vi "FormatDefor.vi"(6 "UnidadesD":u16(ring) caption="Unidades" items=["mm", "inch"], 8 "ValorIn":dbl, 9 "CaptadorD":u16(ring) caption="Captador" items=["Deformación"], 11 "ResoExten":i8(ring) caption="Resolució" items=["0.1", "0.2", "0.5", "0.01", "0.02", "0.05", "0.001", "0.002", "0.005"]) -> (0 "ValorOut":dbl, 3 "NDecimals":u8)   [LabVIEW 2017]
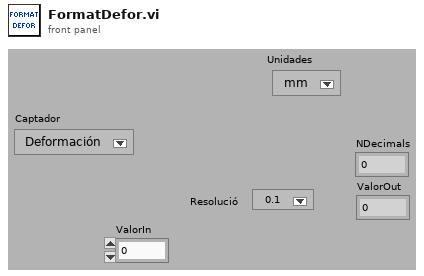
[diagram p1: front panel]
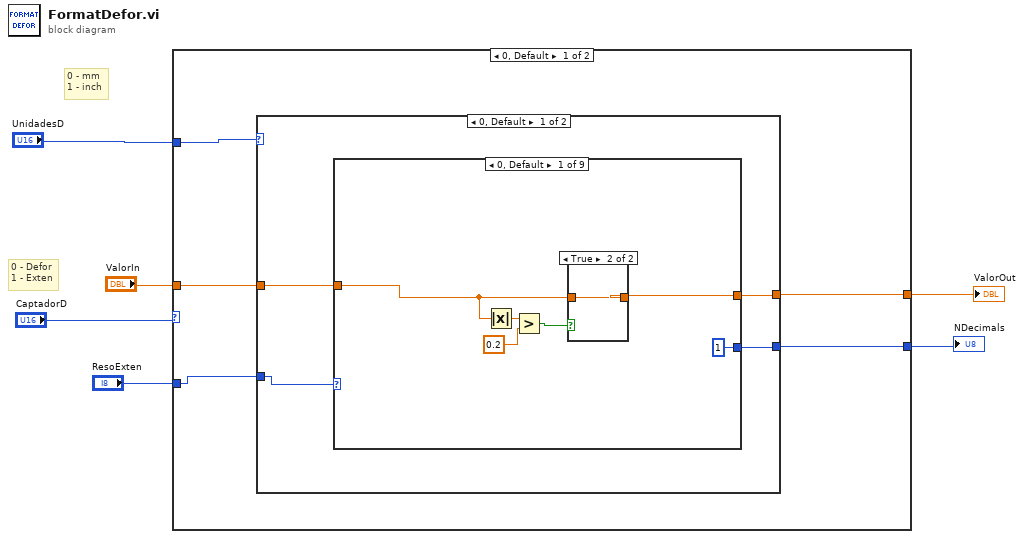
[diagram p0: block diagram]
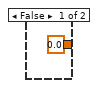
[diagram p2: hidden frame]
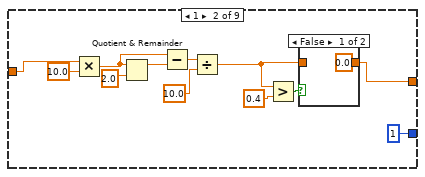
[diagram p3: hidden frame]
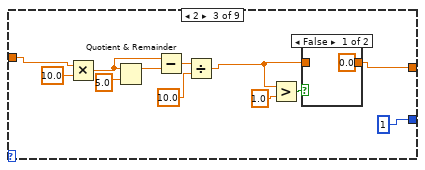
[diagram p5: hidden frame]
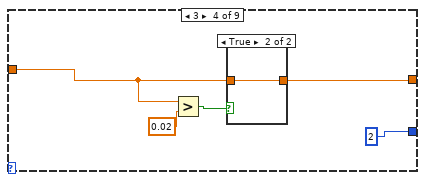
[diagram p7: hidden frame]
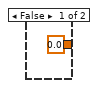
[diagram p8: hidden frame]
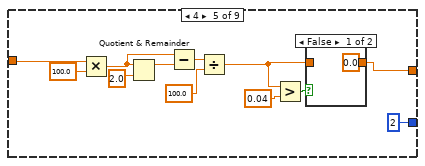
[diagram p9: hidden frame]
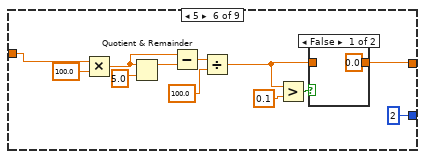
[diagram p11: hidden frame]
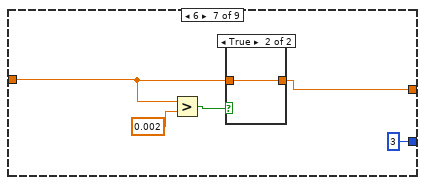
[diagram p13: hidden frame]
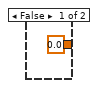
[diagram p14: hidden frame]
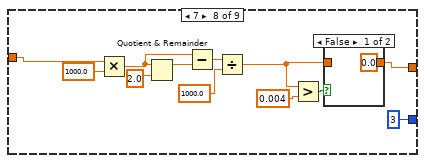
[diagram p15: hidden frame]
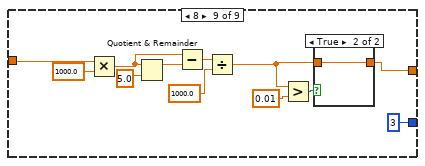
[diagram p17: hidden frame]
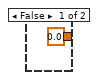
[diagram p18: hidden frame]
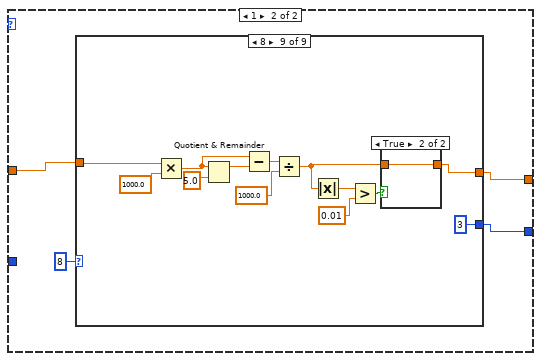
[diagram p19: hidden frame]
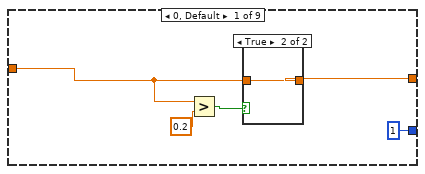
[diagram p20: hidden frame]
diagram:
  # "0 - Defor\n1 - Exten"
  # "0 - mm\n1 - inch"
  n1 = case shown="0, Default" "CaptadorD" {
    tunnel: "ResoExten" -> [w9 w236]
    tunnel: "ValorIn" -> [w10 w235]
    tunnel: [w8 w234] -> w4
    tunnel: [w7 w233] -> w3
    tunnel: "UnidadesD" -> [w11 w232]
    frame 0, Default {
      n2 = case shown="0, Default" w11 {
        tunnel: w10 -> [w13 w125]
        tunnel: w9 -> [w12 _]
        tunnel: [w14 w124] -> w8
        tunnel: [w15 w123] -> w7
        frame 0, Default {
          n3 = case shown="0, Default" w12 {
            tunnel: w13 -> [w18 w25 w40 w54 w61 w74 w89 w95 w110]
            tunnel: [w19 w26 w39 w53 w60 w75 w88 w96 w109] -> w15
            tunnel: [1 ("NDecimals") 1 ("NDecimals") 1 2 ("NDecimals") 2 ("NDecimals") 2 ("NDecimals") 3 ("NDecimals") 3 ("NDecimals") 3 ("NDecimals")] -> w14
            frame 0, Default {
              n4 = Absolute Value(x=w18) -> (abs(x)=w16:dbl)
              n5 = Greater?(x=w16, y=0.2) -> (0:w20:bool)
              n6 = case shown="True" w20 {
                tunnel: w18 -> [_ w23]
                tunnel: [0.0 w23] -> w19
                frame False {
                }
                frame True {
                }
              }
            }
            frame 1 {
              n7 = Multiply(x=w25, y=10.0) -> (x*y=w32:dbl)
              n8 = Quotient & Remainder(x=w32, y=2.0) -> (x-y*floor(x/y)=w33:dbl)  [unwired: 1 out]
              n9 = Subtract(x=w32, y=w33) -> (x-y=w31:dbl)
              n10 = Divide(x=w31, y=10.0) -> (x/y=w27:dbl)
              n11 = Greater?(x=w27, y=0.4) -> (0:w29:bool)
              n12 = case shown="False" w29 {
                tunnel: w27 -> [_ w37]
                tunnel: [0.0 w37] -> w26
                frame False {
                }
                frame True {
                }
              }
            }
            frame 2 {
              n13 = Multiply(x=w40, y=10.0) -> (x*y=w46:dbl)
              n14 = Quotient & Remainder(x=w46, y=5.0) -> (x-y*floor(x/y)=w47:dbl)  [unwired: 1 out]
              n15 = Subtract(x=w46, y=w47) -> (x-y=w45:dbl)
              n16 = Divide(x=w45, y=10.0) -> (x/y=w41:dbl)
              n17 = Greater?(x=w41, y=1.0) -> (0:w43:bool)
              n18 = case shown="False" w43 {
                tunnel: w41 -> [_ w51]
                tunnel: [0.0 w51] -> w39
                frame False {
                }
                frame True {
                }
              }
            }
            frame 3 {
              n19 = Greater?(x=w54, y=0.02) -> (0:w55:bool)
              n20 = case shown="True" w55 {
                tunnel: w54 -> [_ w58]
                tunnel: [0.0 w58] -> w53
                frame False {
                }
                frame True {
                }
              }
            }
            frame 4 {
              n21 = Multiply(x=w61, y=100.0) -> (x*y=w67:dbl)
              n22 = Quotient & Remainder(x=w67, y=2.0) -> (x-y*floor(x/y)=w68:dbl)  [unwired: 1 out]
              n23 = Subtract(x=w67, y=w68) -> (x-y=w66:dbl)
              n24 = Divide(x=w66, y=100.0) -> (x/y=w62:dbl)
              n25 = Greater?(x=w62, y=0.04) -> (0:w64:bool)
              n26 = case shown="False" w64 {
                tunnel: w62 -> [_ w72]
                tunnel: [0.0 w72] -> w60
                frame False {
                }
                frame True {
                }
              }
            }
            frame 5 {
              n27 = Multiply(x=w74, y=100.0) -> (x*y=w81:dbl)
              n28 = Quotient & Remainder(x=w81, y=5.0) -> (x-y*floor(x/y)=w82:dbl)  [unwired: 1 out]
              n29 = Subtract(x=w81, y=w82) -> (x-y=w80:dbl)
              n30 = Divide(x=w80, y=100.0) -> (x/y=w76:dbl)
              n31 = Greater?(x=w76, y=0.1) -> (0:w78:bool)
              n32 = case shown="False" w78 {
                tunnel: w76 -> [_ w86]
                tunnel: [0.0 w86] -> w75
                frame False {
                }
                frame True {
                }
              }
            }
            frame 6 {
              n33 = Greater?(x=w89, y=0.002) -> (0:w90:bool)
              n34 = case shown="True" w90 {
                tunnel: w89 -> [_ w93]
                tunnel: [0.0 w93] -> w88
                frame False {
                }
                frame True {
                }
              }
            }
            frame 7 {
              n35 = Multiply(x=w95, y=1000.0) -> (x*y=w102:dbl)
              n36 = Quotient & Remainder(x=w102, y=2.0) -> (x-y*floor(x/y)=w103:dbl)  [unwired: 1 out]
              n37 = Subtract(x=w102, y=w103) -> (x-y=w101:dbl)
              n38 = Divide(x=w101, y=1000.0) -> (x/y=w97:dbl)
              n39 = Greater?(x=w97, y=0.004) -> (0:w99:bool)
              n40 = case shown="False" w99 {
                tunnel: w97 -> [_ w107]
                tunnel: [0.0 w107] -> w96
                frame False {
                }
                frame True {
                }
              }
            }
            frame 8 {
              n41 = Multiply(x=w110, y=1000.0) -> (x*y=w116:dbl)
              n42 = Quotient & Remainder(x=w116, y=5.0) -> (x-y*floor(x/y)=w117:dbl)  [unwired: 1 out]
              n43 = Subtract(x=w116, y=w117) -> (x-y=w115:dbl)
              n44 = Divide(x=w115, y=1000.0) -> (x/y=w111:dbl)
              n45 = Greater?(x=w111, y=0.01) -> (0:w113:bool)
              n46 = case shown="True" w113 {
                tunnel: w111 -> [_ w121]
                tunnel: [0.0 w121] -> w109
                frame False {
                }
                frame True {
                }
              }
            }
          }
        }
        frame 1 {
          n47 = case shown="8" i8 8 ("ResoExten") {
            tunnel: w125 -> [w127 w134 w149 w163 w170 w183 w198 w204 w220]
            tunnel: [w128 w135 w148 w162 w169 w184 w197 w205 w219] -> w123
            tunnel: [1 ("NDecimals") 1 ("NDecimals") 1 2 ("NDecimals") 2 ("NDecimals") 2 ("NDecimals") 3 ("NDecimals") 3 ("NDecimals") 3 ("NDecimals")] -> w124
            frame 0, Default {
              n48 = Greater?(x=w127, y=0.2) -> (0:w129:bool)
              n49 = case shown="True" w129 {
                tunnel: w127 -> [_ w132]
                tunnel: [0.0 w132] -> w128
                frame False {
                }
                frame True {
                }
              }
            }
            frame 1 {
              n50 = Multiply(x=w134, y=10.0) -> (x*y=w141:dbl)
              n51 = Quotient & Remainder(x=w141, y=2.0) -> (x-y*floor(x/y)=w142:dbl)  [unwired: 1 out]
              n52 = Subtract(x=w141, y=w142) -> (x-y=w140:dbl)
              n53 = Divide(x=w140, y=10.0) -> (x/y=w136:dbl)
              n54 = Greater?(x=w136, y=0.4) -> (0:w138:bool)
              n55 = case shown="False" w138 {
                tunnel: w136 -> [_ w146]
                tunnel: [0.0 w146] -> w135
                frame False {
                }
                frame True {
                }
              }
            }
            frame 2 {
              n56 = Multiply(x=w149, y=10.0) -> (x*y=w155:dbl)
              n57 = Quotient & Remainder(x=w155, y=5.0) -> (x-y*floor(x/y)=w156:dbl)  [unwired: 1 out]
              n58 = Subtract(x=w155, y=w156) -> (x-y=w154:dbl)
              n59 = Divide(x=w154, y=10.0) -> (x/y=w150:dbl)
              n60 = Greater?(x=w150, y=1.0) -> (0:w152:bool)
              n61 = case shown="False" w152 {
                tunnel: w150 -> [_ w160]
                tunnel: [0.0 w160] -> w148
                frame False {
                }
                frame True {
                }
              }
            }
            frame 3 {
              n62 = Greater?(x=w163, y=0.02) -> (0:w164:bool)
              n63 = case shown="True" w164 {
                tunnel: w163 -> [_ w167]
                tunnel: [0.0 w167] -> w162
                frame False {
                }
                frame True {
                }
              }
            }
            frame 4 {
              n64 = Multiply(x=w170, y=100.0) -> (x*y=w176:dbl)
              n65 = Quotient & Remainder(x=w176, y=2.0) -> (x-y*floor(x/y)=w177:dbl)  [unwired: 1 out]
              n66 = Subtract(x=w176, y=w177) -> (x-y=w175:dbl)
              n67 = Divide(x=w175, y=100.0) -> (x/y=w171:dbl)
              n68 = Greater?(x=w171, y=0.04) -> (0:w173:bool)
              n69 = case shown="False" w173 {
                tunnel: w171 -> [_ w181]
                tunnel: [0.0 w181] -> w169
                frame False {
                }
                frame True {
                }
              }
            }
            frame 5 {
              n70 = Multiply(x=w183, y=100.0) -> (x*y=w190:dbl)
              n71 = Quotient & Remainder(x=w190, y=5.0) -> (x-y*floor(x/y)=w191:dbl)  [unwired: 1 out]
              n72 = Subtract(x=w190, y=w191) -> (x-y=w189:dbl)
              n73 = Divide(x=w189, y=100.0) -> (x/y=w185:dbl)
              n74 = Greater?(x=w185, y=0.1) -> (0:w187:bool)
              n75 = case shown="False" w187 {
                tunnel: w185 -> [_ w195]
                tunnel: [0.0 w195] -> w184
                frame False {
                }
                frame True {
                }
              }
            }
            frame 6 {
              n76 = Greater?(x=w198, y=0.002) -> (0:w199:bool)
              n77 = case shown="True" w199 {
                tunnel: w198 -> [_ w202]
                tunnel: [0.0 w202] -> w197
                frame False {
                }
                frame True {
                }
              }
            }
            frame 7 {
              n78 = Multiply(x=w204, y=1000.0) -> (x*y=w211:dbl)
              n79 = Quotient & Remainder(x=w211, y=2.0) -> (x-y*floor(x/y)=w212:dbl)  [unwired: 1 out]
              n80 = Subtract(x=w211, y=w212) -> (x-y=w210:dbl)
              n81 = Divide(x=w210, y=1000.0) -> (x/y=w206:dbl)
              n82 = Greater?(x=w206, y=0.004) -> (0:w208:bool)
              n83 = case shown="False" w208 {
                tunnel: w206 -> [_ w216]
                tunnel: [0.0 w216] -> w205
                frame False {
                }
                frame True {
                }
              }
            }
            frame 8 {
              n84 = Multiply(x=w220, y=1000.0) -> (x*y=w226:dbl)
              n85 = Quotient & Remainder(x=w226, y=5.0) -> (x-y*floor(x/y)=w227:dbl)  [unwired: 1 out]
              n86 = Subtract(x=w226, y=w227) -> (x-y=w225:dbl)
              n87 = Divide(x=w225, y=1000.0) -> (x/y=w221:dbl)
              n88 = Absolute Value(x=w221) -> (abs(x)=w217:dbl)
              n89 = Greater?(x=w217, y=0.01) -> (0:w223:bool)
              n90 = case shown="True" w223 {
                tunnel: w221 -> [_ w231]
                tunnel: [0.0 w231] -> w219
                frame False {
                }
                frame True {
                }
              }
            }
          }
        }
      }
    }
    frame 1 {
      n91 = case shown="1" w232 {
        tunnel: w236 -> [w238 _]
        tunnel: w235 -> [w237 w358]
        tunnel: [w239 w357] -> w234
        tunnel: [w240 w356] -> w233
        frame 0, Default {
          n92 = case shown="8" w238 {
            tunnel: [w244 w252 w267 w282 w290 w305 w320 w328 w343] -> w240
            tunnel: [1 ("NDecimals") 1 ("NDecimals") 1 2 ("NDecimals") 2 ("NDecimals") 2 ("NDecimals") 3 ("NDecimals") 3 ("NDecimals") 3 ("NDecimals")] -> w239
            tunnel: w237 -> [w242 w250 w265 w280 w288 w303 w318 w326 w341]
            frame 0, Default {
              n93 = Absolute Value(x=w242) -> (abs(x)=w241:dbl)
              n94 = Greater?(x=w241, y=0.2) -> (0:w245:bool)
              n95 = case shown="True" w245 {
                tunnel: w242 -> [_ w248]
                tunnel: [0.0 w248] -> w244
                frame False {
                }
                frame True {
                }
              }
            }
            frame 1 {
              n96 = Multiply(x=w250, y=10.0) -> (x*y=w258:dbl)
              n97 = Quotient & Remainder(x=w258, y=2.0) -> (x-y*floor(x/y)=w259:dbl)  [unwired: 1 out]
              n98 = Subtract(x=w258, y=w259) -> (x-y=w257:dbl)
              n99 = Divide(x=w257, y=10.0) -> (x/y=w253:dbl)
              n100 = Absolute Value(x=w253) -> (abs(x)=w249:dbl)
              n101 = Greater?(x=w249, y=0.4) -> (0:w255:bool)
              n102 = case shown="False" w255 {
                tunnel: w253 -> [_ w263]
                tunnel: [0.0 w263] -> w252
                frame False {
                }
                frame True {
                }
              }
            }
            frame 2 {
              n103 = Multiply(x=w265, y=10.0) -> (x*y=w273:dbl)
              n104 = Quotient & Remainder(x=w273, y=5.0) -> (x-y*floor(x/y)=w274:dbl)  [unwired: 1 out]
              n105 = Subtract(x=w273, y=w274) -> (x-y=w272:dbl)
              n106 = Divide(x=w272, y=10.0) -> (x/y=w268:dbl)
              n107 = Absolute Value(x=w268) -> (abs(x)=w264:dbl)
              n108 = Greater?(x=w264, y=1.0) -> (0:w270:bool)
              n109 = case shown="False" w270 {
                tunnel: w268 -> [_ w278]
                tunnel: [0.0 w278] -> w267
                frame False {
                }
                frame True {
                }
              }
            }
            frame 3 {
              n110 = Absolute Value(x=w280) -> (abs(x)=w279:dbl)
              n111 = Greater?(x=w279, y=0.02) -> (0:w283:bool)
              n112 = case shown="True" w283 {
                tunnel: w280 -> [_ w286]
                tunnel: [0.0 w286] -> w282
                frame False {
                }
                frame True {
                }
              }
            }
            frame 4 {
              n113 = Multiply(x=w288, y=100.0) -> (x*y=w296:dbl)
              n114 = Quotient & Remainder(x=w296, y=2.0) -> (x-y*floor(x/y)=w297:dbl)  [unwired: 1 out]
              n115 = Subtract(x=w296, y=w297) -> (x-y=w295:dbl)
              n116 = Divide(x=w295, y=100.0) -> (x/y=w291:dbl)
              n117 = Absolute Value(x=w291) -> (abs(x)=w287:dbl)
              n118 = Greater?(x=w287, y=0.04) -> (0:w293:bool)
              n119 = case shown="False" w293 {
                tunnel: w291 -> [_ w301]
                tunnel: [0.0 w301] -> w290
                frame False {
                }
                frame True {
                }
              }
            }
            frame 5 {
              n120 = Multiply(x=w303, y=100.0) -> (x*y=w311:dbl)
              n121 = Quotient & Remainder(x=w311, y=5.0) -> (x-y*floor(x/y)=w312:dbl)  [unwired: 1 out]
              n122 = Subtract(x=w311, y=w312) -> (x-y=w310:dbl)
              n123 = Divide(x=w310, y=100.0) -> (x/y=w306:dbl)
              n124 = Absolute Value(x=w306) -> (abs(x)=w302:dbl)
              n125 = Greater?(x=w302, y=0.1) -> (0:w308:bool)
              n126 = case shown="False" w308 {
                tunnel: w306 -> [_ w316]
                tunnel: [0.0 w316] -> w305
                frame False {
                }
                frame True {
                }
              }
            }
            frame 6 {
              n127 = Absolute Value(x=w318) -> (abs(x)=w317:dbl)
              n128 = Greater?(x=w317, y=0.002) -> (0:w321:bool)
              n129 = case shown="True" w321 {
                tunnel: w318 -> [_ w324]
                tunnel: [0.0 w324] -> w320
                frame False {
                }
                frame True {
                }
              }
            }
            frame 7 {
              n130 = Multiply(x=w326, y=1000.0) -> (x*y=w334:dbl)
              n131 = Quotient & Remainder(x=w334, y=2.0) -> (x-y*floor(x/y)=w335:dbl)  [unwired: 1 out]
              n132 = Subtract(x=w334, y=w335) -> (x-y=w333:dbl)
              n133 = Divide(x=w333, y=1000.0) -> (x/y=w329:dbl)
              n134 = Absolute Value(x=w329) -> (abs(x)=w325:dbl)
              n135 = Greater?(x=w325, y=0.004) -> (0:w331:bool)
              n136 = case shown="False" w331 {
                tunnel: w329 -> [_ w339]
                tunnel: [0.0 w339] -> w328
                frame False {
                }
                frame True {
                }
              }
            }
            frame 8 {
              n137 = Multiply(x=w341, y=1000.0) -> (x*y=w349:dbl)
              n138 = Quotient & Remainder(x=w349, y=5.0) -> (x-y*floor(x/y)=w350:dbl)  [unwired: 1 out]
              n139 = Subtract(x=w349, y=w350) -> (x-y=w348:dbl)
              n140 = Divide(x=w348, y=1000.0) -> (x/y=w344:dbl)
              n141 = Absolute Value(x=w344) -> (abs(x)=w340:dbl)
              n142 = Greater?(x=w340, y=0.01) -> (0:w346:bool)
              n143 = case shown="True" w346 {
                tunnel: w344 -> [_ w354]
                tunnel: [0.0 w354] -> w343
                frame False {
                }
                frame True {
                }
              }
            }
          }
        }
        frame 1 {
          n144 = case shown="8" i8 8 ("ResoExten") {
            tunnel: w358 -> [w361 w369 w385 w400 w408 w422 w436 w445 w461]
            tunnel: [w362 w370 w384 w399 w407 w423 w438 w446 w460] -> w356
            tunnel: [1 ("NDecimals") 1 ("NDecimals") 1 2 ("NDecimals") 2 ("NDecimals") 2 ("NDecimals") 3 ("NDecimals") 3 ("NDecimals") 3 ("NDecimals")] -> w357
            frame 0, Default {
              n145 = Absolute Value(x=w361) -> (abs(x)=w359:dbl)
              n146 = Greater?(x=w359, y=0.2) -> (0:w363:bool)
              n147 = case shown="True" w363 {
                tunnel: w361 -> [_ w366]
                tunnel: [0.0 w366] -> w362
                frame False {
                }
                frame True {
                }
              }
            }
            frame 1 {
              n148 = Multiply(x=w369, y=10.0) -> (x*y=w376:dbl)
              n149 = Quotient & Remainder(x=w376, y=2.0) -> (x-y*floor(x/y)=w377:dbl)  [unwired: 1 out]
              n150 = Subtract(x=w376, y=w377) -> (x-y=w375:dbl)
              n151 = Divide(x=w375, y=10.0) -> (x/y=w371:dbl)
              n152 = Absolute Value(x=w371) -> (abs(x)=w367:dbl)
              n153 = Greater?(x=w367, y=0.4) -> (0:w373:bool)
              n154 = case shown="False" w373 {
                tunnel: w371 -> [_ w381]
                tunnel: [0.0 w381] -> w370
                frame False {
                }
                frame True {
                }
              }
            }
            frame 2 {
              n155 = Multiply(x=w385, y=10.0) -> (x*y=w391:dbl)
              n156 = Quotient & Remainder(x=w391, y=5.0) -> (x-y*floor(x/y)=w392:dbl)  [unwired: 1 out]
              n157 = Subtract(x=w391, y=w392) -> (x-y=w390:dbl)
              n158 = Divide(x=w390, y=10.0) -> (x/y=w386:dbl)
              n159 = Absolute Value(x=w386) -> (abs(x)=w382:dbl)
              n160 = Greater?(x=w382, y=1.0) -> (0:w388:bool)
              n161 = case shown="False" w388 {
                tunnel: w386 -> [_ w396]
                tunnel: [0.0 w396] -> w384
                frame False {
                }
                frame True {
                }
              }
            }
            frame 3 {
              n162 = Absolute Value(x=w400) -> (abs(x)=w397:dbl)
              n163 = Greater?(x=w397, y=0.02) -> (0:w401:bool)
              n164 = case shown="True" w401 {
                tunnel: w400 -> [_ w404]
                tunnel: [0.0 w404] -> w399
                frame False {
                }
                frame True {
                }
              }
            }
            frame 4 {
              n165 = Multiply(x=w408, y=100.0) -> (x*y=w414:dbl)
              n166 = Quotient & Remainder(x=w414, y=2.0) -> (x-y*floor(x/y)=w415:dbl)  [unwired: 1 out]
              n167 = Subtract(x=w414, y=w415) -> (x-y=w413:dbl)
              n168 = Divide(x=w413, y=100.0) -> (x/y=w409:dbl)
              n169 = Absolute Value(x=w409) -> (abs(x)=w405:dbl)
              n170 = Greater?(x=w405, y=0.04) -> (0:w411:bool)
              n171 = case shown="False" w411 {
                tunnel: w409 -> [_ w419]
                tunnel: [0.0 w419] -> w407
                frame False {
                }
                frame True {
                }
              }
            }
            frame 5 {
              n172 = Multiply(x=w422, y=100.0) -> (x*y=w429:dbl)
              n173 = Quotient & Remainder(x=w429, y=5.0) -> (x-y*floor(x/y)=w430:dbl)  [unwired: 1 out]
              n174 = Subtract(x=w429, y=w430) -> (x-y=w428:dbl)
              n175 = Divide(x=w428, y=100.0) -> (x/y=w424:dbl)
              n176 = Absolute Value(x=w424) -> (abs(x)=w420:dbl)
              n177 = Greater?(x=w420, y=0.1) -> (0:w426:bool)
              n178 = case shown="False" w426 {
                tunnel: w424 -> [_ w434]
                tunnel: [0.0 w434] -> w423
                frame False {
                }
                frame True {
                }
              }
            }
            frame 6 {
              n179 = Absolute Value(x=w436) -> (abs(x)=w435:dbl)
              n180 = Greater?(x=w435, y=0.002) -> (0:w439:bool)
              n181 = case shown="True" w439 {
                tunnel: w436 -> [_ w442]
                tunnel: [0.0 w442] -> w438
                frame False {
                }
                frame True {
                }
              }
            }
            frame 7 {
              n182 = Multiply(x=w445, y=1000.0) -> (x*y=w452:dbl)
              n183 = Quotient & Remainder(x=w452, y=2.0) -> (x-y*floor(x/y)=w453:dbl)  [unwired: 1 out]
              n184 = Subtract(x=w452, y=w453) -> (x-y=w451:dbl)
              n185 = Divide(x=w451, y=1000.0) -> (x/y=w447:dbl)
              n186 = Absolute Value(x=w447) -> (abs(x)=w443:dbl)
              n187 = Greater?(x=w443, y=0.004) -> (0:w449:bool)
              n188 = case shown="False" w449 {
                tunnel: w447 -> [_ w457]
                tunnel: [0.0 w457] -> w446
                frame False {
                }
                frame True {
                }
              }
            }
            frame 8 {
              n189 = Multiply(x=w461, y=1000.0) -> (x*y=w467:dbl)
              n190 = Quotient & Remainder(x=w467, y=5.0) -> (x-y*floor(x/y)=w468:dbl)  [unwired: 1 out]
              n191 = Subtract(x=w467, y=w468) -> (x-y=w466:dbl)
              n192 = Divide(x=w466, y=1000.0) -> (x/y=w462:dbl)
              n193 = Absolute Value(x=w462) -> (abs(x)=w458:dbl)
              n194 = Greater?(x=w458, y=0.01) -> (0:w464:bool)
              n195 = case shown="True" w464 {
                tunnel: w462 -> [_ w472]
                tunnel: [0.0 w472] -> w460
                frame False {
                }
                frame True {
                }
              }
            }
          }
        }
      }
    }
  }
  "ValorOut" <- w3
  "NDecimals" <- w4
